vi "test Signed and Unsigned.vi"(8 "error in (no error)":errorcluster, 11 "TestCase in":refnum<class "BNR.lvclass">) -> (0 "error out":errorcluster, 3 "TestCase out":refnum<class "BNR.lvclass">)   [LabVIEW 2027, in "BNR.lvclass"]
uses:
  BNR.lvclass
  52a9e853-f441-4a14-a3ae-af5dd9b478de.vi
  fabf7f84-3cd3-4adf-92be-b1484a105bea.vi
  1abdb739-fb66-4f21-b2ba-a9918976e5c4.vi
  65c3b74b-7b29-4765-ab7a-f8a38be437e9.vi
  4bb312ad-4e10-4980-9d7d-1c2267be8d4c.vi
  24d2de50-4032-47ef-a2ca-660952972ed8.vi
  52a9e853-f441-4a14-a3ae-af5dd9b478de.vi/9377bb8f-44b5-4a8f-87f1-966fd5a9edcc.vi
  52a9e853-f441-4a14-a3ae-af5dd9b478de.vi/e95d9d1f-307c-44d6-9f26-c3f519a4990d.vi
  52a9e853-f441-4a14-a3ae-af5dd9b478de.vi/0c23f515-4369-4514-bc3d-4444e6b437b2.vi
  fabf7f84-3cd3-4adf-92be-b1484a105bea.vi/9377bb8f-44b5-4a8f-87f1-966fd5a9edcc.vi
  fabf7f84-3cd3-4adf-92be-b1484a105bea.vi/e95d9d1f-307c-44d6-9f26-c3f519a4990d.vi
  fabf7f84-3cd3-4adf-92be-b1484a105bea.vi/0c23f515-4369-4514-bc3d-4444e6b437b2.vi
  1abdb739-fb66-4f21-b2ba-a9918976e5c4.vi/16a2565b-3c16-407b-a626-9da2a3da432e.vi
  65c3b74b-7b29-4765-ab7a-f8a38be437e9.vi/9377bb8f-44b5-4a8f-87f1-966fd5a9edcc.vi
  65c3b74b-7b29-4765-ab7a-f8a38be437e9.vi/e95d9d1f-307c-44d6-9f26-c3f519a4990d.vi
  65c3b74b-7b29-4765-ab7a-f8a38be437e9.vi/0c23f515-4369-4514-bc3d-4444e6b437b2.vi
  4bb312ad-4e10-4980-9d7d-1c2267be8d4c.vi/16a2565b-3c16-407b-a626-9da2a3da432e.vi
  24d2de50-4032-47ef-a2ca-660952972ed8.vi/9377bb8f-44b5-4a8f-87f1-966fd5a9edcc.vi
  24d2de50-4032-47ef-a2ca-660952972ed8.vi/e95d9d1f-307c-44d6-9f26-c3f519a4990d.vi
  24d2de50-4032-47ef-a2ca-660952972ed8.vi/0c23f515-4369-4514-bc3d-4444e6b437b2.vi
  C:/Program Files/National Instruments/LabVIEW 2027/vi.lib/addons/_JKI Toolkits/VI Tester/TestCase.llb/TestCase.lvclass
  <vilib>/addons/_JKI Toolkits/VI Tester/TestCase.llb/TestCase.lvclass
panel:
  out "BNR encoded value":bool[](array[boolean])
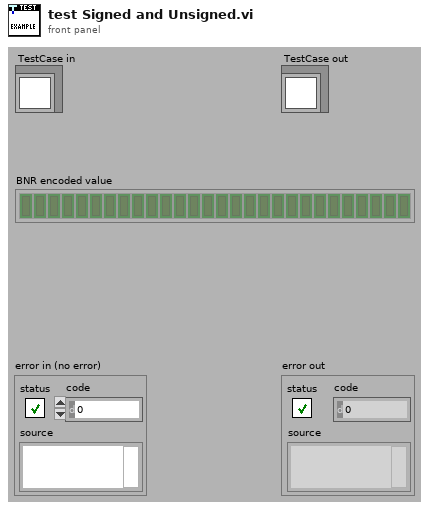
[diagram p1: front panel]
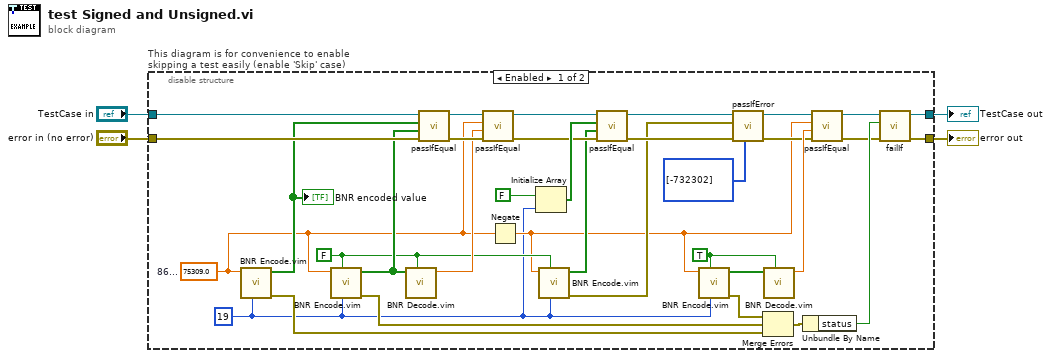
[diagram p0: block diagram]
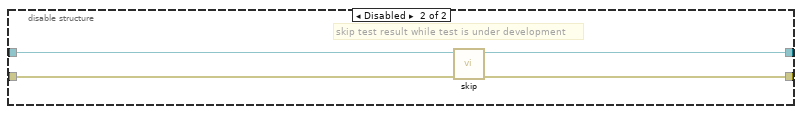
[diagram p2: hidden frame]
diagram:
  n1 = disable-structure "This diagram is for convenience to enable skipping a test easily (enable 'Skip' case)" shown="Enabled" {
    disable-tunnel: "TestCase in" -> [w37 w42]
    disable-tunnel: [w29 w40] -> w2
    disable-tunnel: [w30 w41] -> w1
    disable-tunnel: "error in (no error)" -> [w35 w39]
    frame Enabled {
      w8 = TRUE ("signed")
      w9 = FALSE ("signed")
      w6 = 19 ("data size (bits)")
      w5 = 75309.0  # 86...
      n2 = call "BNR Encode.vim"("data size (bits)"=w6, "value"=w5) -> ("error out"=w28:errorcluster, "BNR encoded value"=w21:bool[])  [unwired: 8 in]
      "BNR encoded value" <- w21
      n3 = call "BNR Encode.vim"("data size (bits)"=w6, "signed"=w9, "value"=w5) -> ("error out"=w27:errorcluster, "BNR encoded value"=w23:bool[])  [unwired: 7 in]
      n4 = call "BNR Decode.vim"("signed"=w9, "BNR encoded value"=w23) -> ("value"=w22:dbl)  [unwired: 9 in]
      n5 = call-dynamic "passIfEqual.vi"("error in (no error)"=w35, "y"=w23, "x"=w21, "TestCase in"=w37) -> ("error out"=w36:errorcluster, "TestCase out"=w38:refnum<class "BNR.lvclass">)  [unwired: 6 in]
      n6 = call-dynamic "passIfEqual.vi"("error in (no error)"=w36, "y"=w22, "x"=w5, "TestCase in"=w38) -> ("error out"=w14:errorcluster, "TestCase out"=w15:refnum<class "BNR.lvclass">)  [unwired: 6 in]
      n7 = Negate(x=w5) -> (-x=w7:dbl)
      n8 = Initialize Array(FALSE ("signed"), w6) -> (w16:bool[])
      n9 = call "BNR Encode.vim"("data size (bits)"=w6, "signed"=w9, "value"=w7) -> ("error out"=w10:errorcluster, "BNR encoded value"=w11:bool[])  [unwired: 7 in]
      n10 = call-dynamic "passIfEqual.vi"("error in (no error)"=w14, "y"=w11, "x"=w16, "TestCase in"=w15) -> ("error out"=w19:errorcluster, "TestCase out"=w20:refnum<class "BNR.lvclass">)  [unwired: 6 in]
      n11 = call "BNR Encode.vim"("data size (bits)"=w6, "signed"=w8, "value"=w7) -> ("error out"=w26:errorcluster, "BNR encoded value"=w25:bool[])  [unwired: 7 in]
      n12 = call-dynamic "passIfError.vi"("passing error codes (default = any error code)"=i32[] [-732302], "error in (no error)"=w19, "error"=w10, "TestCase in"=w20) -> ("error out"=w12:errorcluster, "TestCase out"=w13:refnum<class "BNR.lvclass">)  [unwired: 6 in]
      n13 = Merge Errors(w26, w27, w28) -> (w34:errorcluster)
      n14 = call "BNR Decode.vim"("signed"=w8, "BNR encoded value"=w25) -> ("value"=w24:dbl)  [unwired: 9 in]
      n15 = Unbundle By Name(w34) -> ("status"=w33:bool)
      n16 = call-dynamic "passIfEqual.vi"("error in (no error)"=w12, "y"=w24, "x"=w7, "TestCase in"=w13) -> ("error out"=w31:errorcluster, "TestCase out"=w32:refnum<class "BNR.lvclass">)  [unwired: 6 in]
      n17 = call-dynamic "failIf.vi"("error in (no error)"=w31, "fail"=w33, "TestCase in"=w32) -> ("error out"=w30:errorcluster, "TestCase out"=w29:refnum<class "BNR.lvclass">)  [unwired: 7 in]
    }
    frame Disabled {
      # "skip test result while test is under development"
      n18 = call <vilib>:"skip.vi"("error in (no error)"=w39, "TestCase in"=w42) -> ("error out"=w41:errorcluster, "TestCase out"=w40:refnum<class "BNR.lvclass">)  [unwired: 8 in]
    }
  }
  "error out" <- w1
  "TestCase out" <- w2
